vi "microFPGA_camera_swstart_trigger_addr_41_ctrl.vi"(0 "VISA resource name":refnum<visa-resource-name>, 2 "write or read":u16(ring) items=["read", "write"], 5 "Camera_sw_start_WRITE":u16(ring) items=["Stop = 0", "Start = 1 "], 11 "error in (no error)":errorcluster) -> (4 "VISA resource name 2":refnum<visa-resource-name>, 6 "Camera_sw_start_READ":u16(ring) items=["Stop = 0", "Start = 1 "], 8 "value write confirm":bool, 10 "abort_wrong_input":bool, 15 "error out":errorcluster)   [LabVIEW 2021]
panel:
  out "mode read string answer":string
  out "mode read string":string
  out "mode write string":string
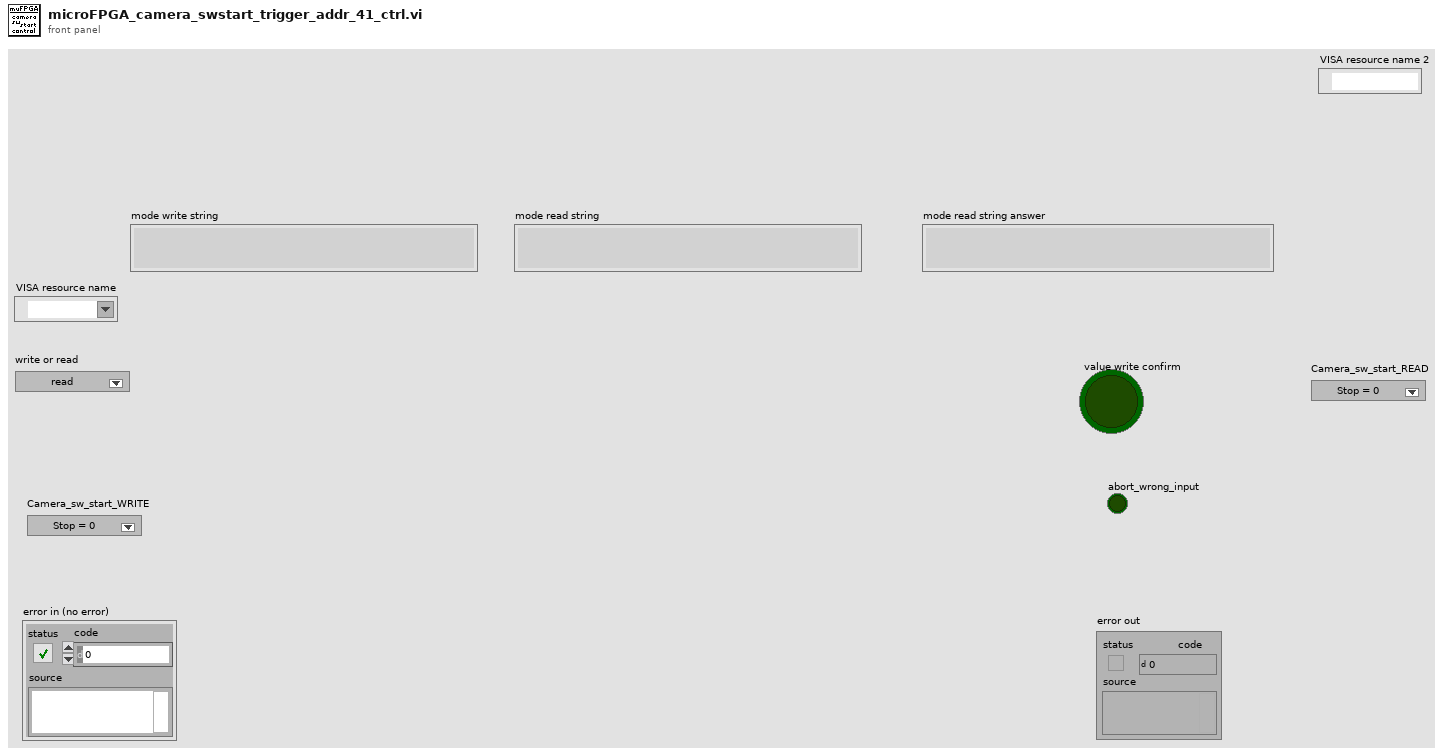
[diagram p1: front panel]
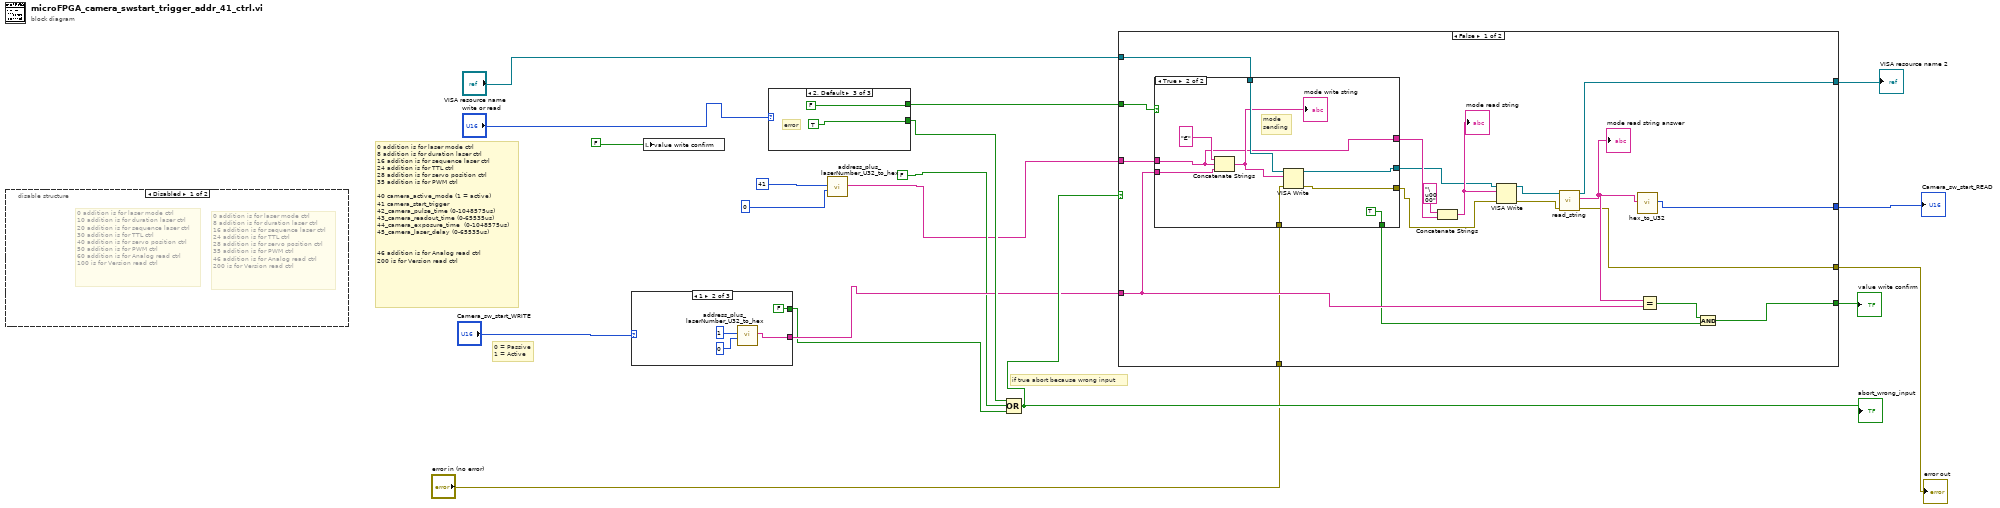
[diagram p0: block diagram]
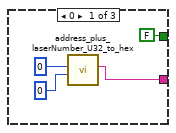
[diagram p3: hidden frame]
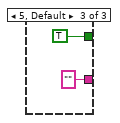
[diagram p4: hidden frame]
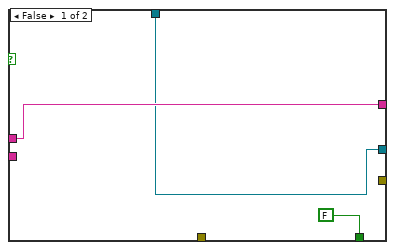
[diagram p5: hidden frame]
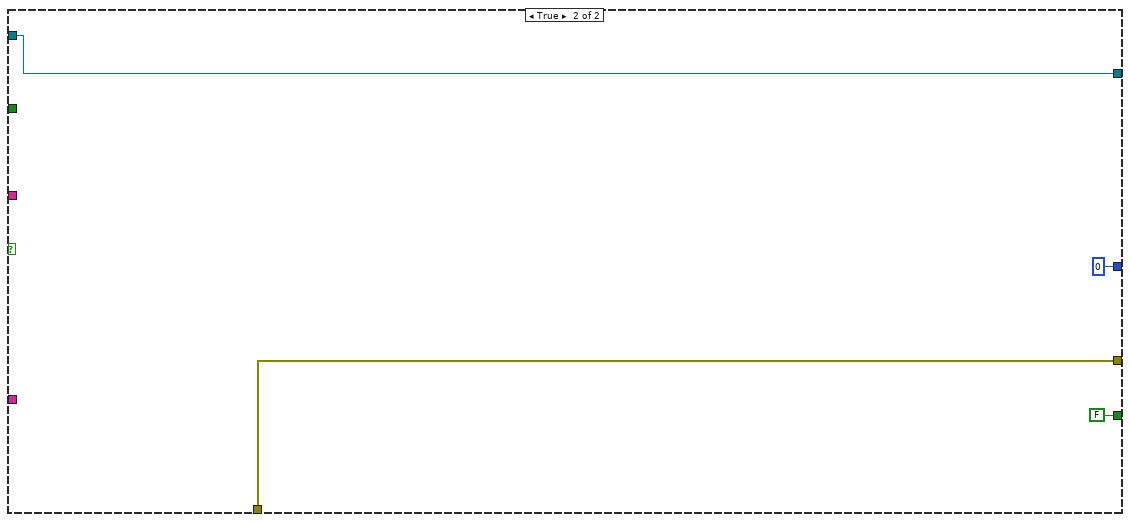
[diagram p6: hidden frame]
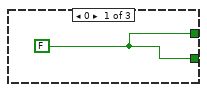
[diagram p7: hidden frame]
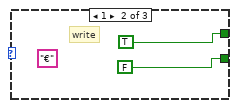
[diagram p8: hidden frame]
diagram:
  # "0 addition is for laser mode ctrl\n8 addition is for duration laser ctrl\n16 addition is for sequence laser ctrl\n24 addition is for TTL ctrl\n28 addition is for servo position ctrl\n35 addition is for PWM ctrl\n\n40 camera_active_mode (1 = active) \n41 camera_start_trigger\n42_camera_pulse_time (0-1048575us)\n43_camera_readout_time (0-65535us)\n44_camera_exposure_time  (0-1048575us)\n45_camera_laser_delay (0-65535us)\n\n\n46 addition is for Analog read ctrl\n200 is for Version read ctrl"
  # "0 = Passive\n1 = Active"
  # "if true abort because wrong input"
  n1 = disable-structure shown="Disabled" {
    frame Disabled {
      # "0 addition is for laser mode ctrl\n8 addition is for duration laser ctrl\n16 addition is for sequence laser ctrl\n24 addition is for TTL ctrl\n28 addition is for servo position ctrl\n35 addition is for PWM ctrl\n46 addition is for Analog read ctrl\n200 is for Version read ctrl"
      # "0 addition is for laser mode ctrl\n10 addition is for duration laser ctrl\n20 addition is for sequence laser ctrl\n30 addition is for TTL ctrl\n40 addition is for servo position ctrl\n50 addition is for PWM ctrl\n60 addition is for Analog read ctrl\n100 is for Version read ctrl"
    }
    frame Enabled {
    }
  }
  n2 = case shown="1" "Camera_sw_start_WRITE" {
    tunnel: [w19 w24 "" ("string 5")] -> w7
    tunnel: [FALSE FALSE TRUE] -> w6
    frame 0 {
      n3 = call "address_plus_laserNumber_U32_to_hex.vi"("adress offset"=u32 0, "y 3"=u32 0) -> ("string 5"=w19:string)  [unwired: 8 in]
    }
    frame 1 {
      n4 = call "address_plus_laserNumber_U32_to_hex.vi"("adress offset"=u32 0, "y 3"=u32 1) -> ("string 5"=w24:string)  [unwired: 8 in]
    }
    frame 5, Default {
    }
  }
  n5 = local write "value write confirm"(FALSE ("value confirm")) -> ()
  n6 = case shown="2, Default" "write or read" {
    tunnel: [w29 TRUE FALSE] -> w16
    tunnel: [w29 FALSE TRUE] -> w14
    frame 0 {
      w29 = FALSE
    }
    frame 1 {
      (unwired) "€" ("hex")
      # "write"
    }
    frame 2, Default {
      # "error"
    }
  }
  n7 = call "address_plus_laserNumber_U32_to_hex.vi"("adress offset"=u32 0, "y 3"=u32 41) -> ("string 5"=w3:string)  [unwired: 8 in]
  n8 = Compound Arithmetic op=OR(w14, FALSE, w6) -> (w12:bool)
  "abort_wrong_input" <- w12
  n9 = case shown="False" w12 {
    tunnel: "VISA resource name" -> [w52 w66]
    tunnel: w3 -> [w49 _]
    tunnel: w16 -> [w43 _]
    tunnel: w7 -> [w41 _]
    tunnel: [w40 u32 0 ("U32")] -> w1
    tunnel: [w34 FALSE] -> w13
    tunnel: [w39 w66] -> w11
    tunnel: "error in (no error)" -> [w38 w65]
    tunnel: [w37 w65] -> w9
    frame False {
      n10 = case shown="True" w43 {
        tunnel: w49 -> [w55 w61]
        tunnel: w52 -> [w54 w63]
        tunnel: [w55 w61] -> w50
        tunnel: w41 -> [_ w60]
        tunnel: [w54 w59] -> w45
        tunnel: [_ w58] -> w44
        tunnel: w38 -> [_ w57]
        tunnel: [FALSE TRUE] -> w36
        frame False {
        }
        frame True {
          # "mode \nsending"
          n11 = Concatenate Strings("€" ("string"), w61, w60) -> (w62:string)
          "mode write string" <- w62
          n12 = VISA Write(VISA resource name=w63, write buffer=w62, error in (no error)=w57) -> (VISA resource name out=w59:refnum<visa-resource-name>, error out=w58:errorcluster)  [unwired: 1 out]
        }
      }
      n13 = Concatenate Strings("\u0000" ("string"), w50) -> (w48:string)
      "mode read string" <- w48
      n14 = VISA Write(VISA resource name=w45, write buffer=w48, error in (no error)=w44) -> (VISA resource name out=w47:refnum<visa-resource-name>, error out=w46:errorcluster)  [unwired: 1 out]
      n15 = call "read_string.vi"("error in (no error)"=w46, "VISA resource name 2"=w47) -> ("error out"=w37:errorcluster, "read buffer"=w42:string, "VISA resource name"=w39:refnum<visa-resource-name>)  [unwired: 7 in]
      "mode read string answer" <- w42
      n16 = call "hex_to_U32.vi"("hex"=w42) -> ("U32"=w40:u32)  [unwired: 9 in]
      n17 = Equal?(x=w42, y=w41) -> (x = y?=w35:bool)
      n18 = And(x=w35, y=w36) -> (x .and. y?=w34:bool)
    }
    frame True {
    }
  }
  "value write confirm" <- w13
  "VISA resource name 2" <- w11
  "error out" <- w9
  "Camera_sw_start_READ" <- w1
